vi "Cycle through Scrollable Strings.vi"(6 "Stop?":T1, 9 "Scroll Interval":T2, 10 "Scrollable Messages Array Size":i32, 11 "Scrolling Messages Array":string[](array[string])) -> (3 "String to Display":T3)   [LabVIEW 2021]
uses:
  <extravilib>/ChannelInstances/Stream-str/)Channel.ctl
  <extravilib>/ChannelInstances/Tag-u32/))Channel.ctl
  <extravilib>/ChannelInstances/Tag-bool/))Channel.ctl
  <extravilib>/ChannelInstances/Tag-u32/Read With Abort.vi
  <extravilib>/ChannelInstances/Tag-bool/Read With Abort.vi
  <extravilib>/ChannelInstances/Stream-str/Write With Abort.vi
  <extravilib>/ChannelInstances/Stream-str/Endpoint.vi
  <extravilib>/ChannelInstances/Tag-u32/EndpointRead.vi
  <extravilib>/ChannelInstances/Tag-bool/EndpointRead.vi
  <extravilib>/ChannelInstances/Stream-str/)Channel.vi
  <resource>/ChannelSupport/_ChannelSupport/WaitIfNeeded.vi
  <extravilib>/ChannelInstances/Tag-bool.lvlib
  <extravilib>/ChannelInstances/Tag-u32.lvlib
  <extravilib>/ChannelInstances/Stream-str.lvlib
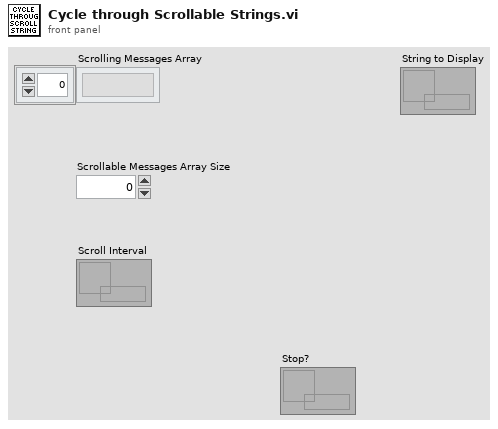
[diagram p1: front panel]
types:
  T1 = typedef "Tag-bool.lvlib/))Channel.ctl" = refnum<queue>
  T2 = typedef "Tag-u32.lvlib/))Channel.ctl" = refnum<queue>
  T3 = typedef "Stream-str.lvlib/)Channel.ctl" = refnum<queue>
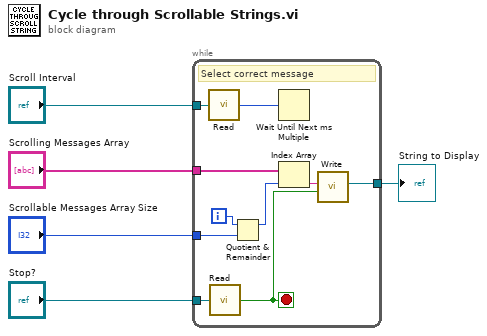
[diagram p0: block diagram]
diagram:
  n1 = while {
    tunnel: "Scrolling Messages Array" -> [w15]
    tunnel: "Scrollable Messages Array Size" -> [w13]
    tunnel: "Stop?" -> [w11]
    tunnel: "Scroll Interval" -> [w10]
    tunnel: [w6] -> w5
    i -> [w14]
    stop <- w7 stop-if-true
    # "Select correct message"
    n2 = call <extravilib>:"Read.vi"("channel"=w10) -> ("element"=w9:u32)  [unwired: 1 in, 1 out]
    n3 = call <extravilib>:"Read.vi"("channel"=w11) -> ("element"=w7:bool)  [unwired: 1 in, 1 out]
    n4 = Quotient & Remainder(x=w14, y=w13) -> (x-y*floor(x/y)=w12:i32)  [unwired: 1 out]
    n5 = Wait Until Next ms Multiple(millisecond multiple=w9) -> ()  [unwired: 1 out]
    n6 = Index Array(array=w15, index=w12) -> (element=w8:string)
    n7 = call <extravilib>:"Write.vi"("last element? (F)"=w7, "element"=w8) -> ("channel"=w6:T3)  [unwired: 7 in, 2 out]
  }
  "String to Display" <- w5
